vi "svx_Continuous Swept-Sine Waveform.vi"(10 "block size [samples]":i32, 11 "chirp settings":T1={"amplitude"=0.0, "frequency range"={"start (Hz)"=20.0, "stop (Hz)"=20000.0, "frequency spacing"=enum."Logarithmic"}, "sampling info"={"Fs"=50000.0, "chirp duration [s]"=3.0}, "initial states"={"frequency [Hz]"=20.0, "phase [rad]"=0.0, "elapsed time [s]"=0.0}, "frequency slope"=0.0, "maximum harmonic"=0, "prefix len [samples]"={"integer"=0, "fractional"=0.0}} {"frequency slope" format="%.2f"; "prefix len [samples]"."fractional" format="%.2p"; "initial states"."elapsed time [s]" format="%.2f"; "initial states"."phase [rad]" format="%.2f"; "initial states"."frequency [Hz]" format="%.2f"; "sampling info"."chirp duration [s]" format="%.2f"; "sampling info"."Fs" format="%.2p"; "frequency range"."stop (Hz)" format="%.2f"; "frequency range"."start (Hz)" format="%.2f"; "amplitude" format="%.2f"}) -> (1 "end reached?":bool, 2 "chirp signal":dbl[](array[numeric]), 3 "chirp settings out":T1={"amplitude"=0.0, "frequency range"={"start (Hz)"=20.0, "stop (Hz)"=20000.0, "frequency spacing"=enum."Logarithmic"}, "sampling info"={"Fs"=50000.0, "chirp duration [s]"=3.0}, "initial states"={"frequency [Hz]"=20.0, "phase [rad]"=0.0, "elapsed time [s]"=0.0}, "frequency slope"=0.0, "maximum harmonic"=0, "prefix len [samples]"={"integer"=0, "fractional"=0.0}} {"frequency slope" format="%.2f"; "prefix len [samples]"."fractional" format="%.2p"; "initial states"."elapsed time [s]" format="%.2f"; "initial states"."phase [rad]" format="%.2f"; "initial states"."frequency [Hz]" format="%.2f"; "sampling info"."chirp duration [s]" format="%.2f"; "sampling info"."Fs" format="%.2p"; "frequency range"."stop (Hz)" format="%.2f"; "frequency range"."start (Hz)" format="%.2f"; "amplitude" format="%.2f"})   [LabVIEW 2017]
uses:
  <vilib>/addons/_NISVFA/_Generation/subVIs/sv_Chirp Settings.ctl
  <vilib>/Analysis/1siggen.llb/Ramp Pattern by Samples.vi
  <vilib>/addons/_NISVFA/_Generation/SoundVib_Generation.lvlib
  <vilib>/Analysis/NI_AALBase.lvlib
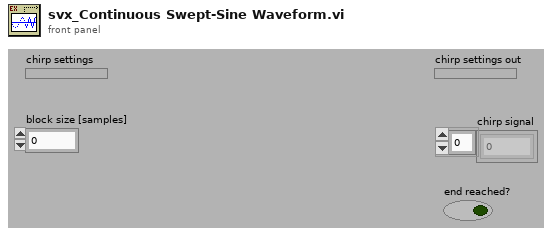
[diagram p1: front panel]
types:
  T1 = typedef "SoundVib_Generation.lvlib/sv_Chirp Settings.ctl" = cluster{"amplitude":dbl, "frequency range":cluster{"start (Hz)":dbl, "stop (Hz)":dbl, "frequency spacing":enum16{"Linear", "Logarithmic"}}, "sampling info":cluster{"Fs":dbl, "chirp duration [s]":dbl}, "initial states":cluster{"frequency [Hz]":dbl, "phase [rad]":dbl, "elapsed time [s]":dbl}, "frequency slope":dbl, "maximum harmonic":i32, "prefix len [samples]":cluster{"integer":u32, "fractional":dbl}}
  T2 = cluster{"frequency [Hz]":dbl, "phase [rad]":dbl, "elapsed time [s]":dbl}
  T3 = cluster{"start (Hz)":dbl, "stop (Hz)":dbl, "frequency spacing":enum16{"Linear", "Logarithmic"}}
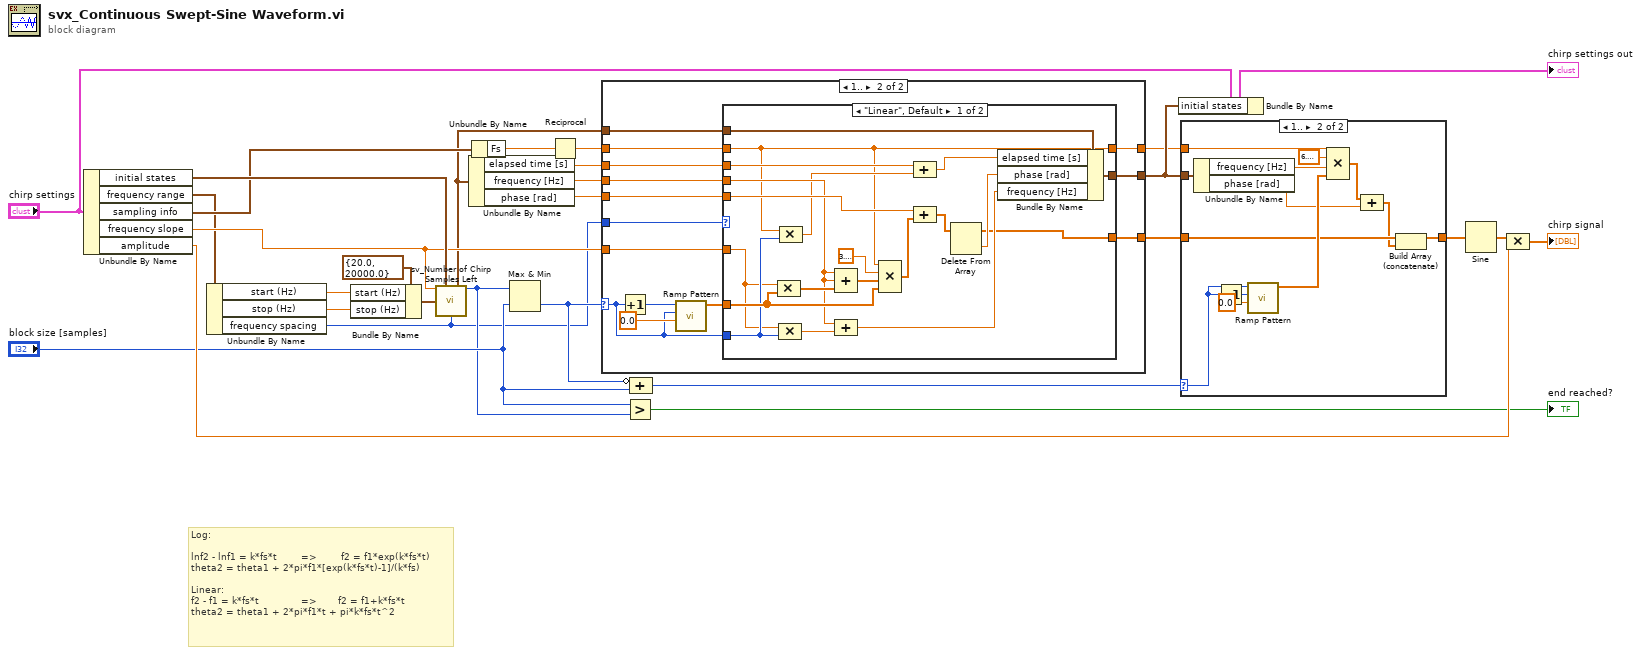
[diagram p0: block diagram]
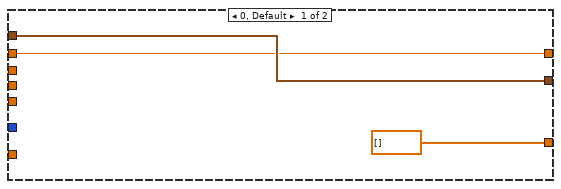
[diagram p2: hidden frame]
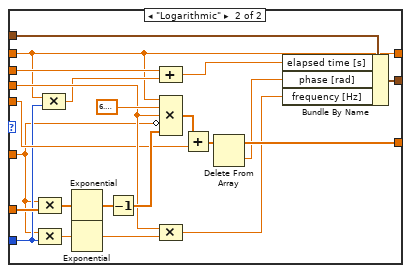
[diagram p3: hidden frame]
diagram:
  # "Log:\n            \nlnf2 - lnf1 = k*fs*t        =>        f2 = f1*exp(k*fs*t)\ntheta2 = theta1 + 2*pi*f1*[exp(k*fs*t)-1]/(k*fs)\n\nLinear:\nf2 - f1 = k*fs*t              =>       f2 = f1+k*fs*t\ntheta2 = theta1 + 2*pi*f1*t + pi*k*fs*t^2"
  n1 = Unbundle By Name("chirp settings") -> ("initial states"=w29:T2, "frequency range"=w9:T3, "sampling info"=w28:cluster{"Fs":dbl, "chirp duration [s]":dbl}, "frequency slope"=w27:dbl, "amplitude"=w15:dbl)
  n2 = Unbundle By Name(w9) -> ("start (Hz)"=w7:dbl, "stop (Hz)"=w6:dbl, "frequency spacing"=w1:enum16{"Linear", "Logarithmic"})
  n3 = Bundle By Name(cluster=cluster{"start (Hz)":dbl, "stop (Hz)":dbl} {"start (Hz)"=20.0, "stop (Hz)"=20000.0} ("frequency range"), "start (Hz)"=w7, "stop (Hz)"=w6) -> (w5:cluster{"start (Hz)":dbl, "stop (Hz)":dbl})
  n4 = call <vilib>:"sv_Number of Chirp Samples Left.vi"("frequency slope"=w27, "initial states"=w29, "frequency range"=w5, "frequency spacing"=w1) -> ("initial states out"=w22:T2, "# of samples left"=w3:i32)  [unwired: 9 in, 1 out]
  n5 = Unbundle By Name(w22) -> ("elapsed time [s]"=w23:dbl, "frequency [Hz]"=w26:dbl, "phase [rad]"=w25:dbl)
  n6 = Unbundle By Name(w28) -> ("Fs"=w24:dbl)
  n7 = Max & Min(x=w3, y="block size [samples]") -> (min(x,y)=w12:i32)  [unwired: 1 out]
  n8 = Reciprocal(x=w24) -> (1/x=w21:dbl)
  n9 = case shown="1.." w12 {
    selector: w12 -> [_ w33]
    tunnel: w27 -> [_ w46]
    tunnel: w26 -> [_ w45]
    tunnel: w25 -> [_ w44]
    tunnel: w1 -> [_ w40]
    tunnel: [dbl[] [] w39] -> w11
    tunnel: w23 -> [_ w38]
    tunnel: w22 -> [w32 w37]
    tunnel: w21 -> [w31 w36]
    tunnel: [w32 w35] -> w17
    tunnel: [w31 w34] -> w16
    frame 0, Default {
    }
    frame 1.. {
      n10 = Increment(x=w33) -> (x+1=w42:i32)
      n11 = call-poly <vilib>:"Ramp Pattern.vi"("start"=0.0, "end"=w33, "samples"=w42) -> ("Ramp Pattern"=w41:dbl[])  [unwired: 7 in, 1 out]
      n12 = case shown="\"Linear\", Default" w40 {
        tunnel: w45 -> [w56 w79]
        tunnel: w44 -> [w63 w76]
        tunnel: w46 -> [w48 w70]
        tunnel: w41 -> [w64 w84]
        tunnel: w37 -> [w49 w71]
        tunnel: w33 -> [w53 w75]
        tunnel: [w60 w78] -> w35
        tunnel: w36 -> [w47 w67]
        tunnel: [w54 w77] -> w39
        tunnel: w38 -> [w51 w73]
        tunnel: [w47 w67] -> w34
        frame "Linear", Default {
          n13 = Compound Arithmetic op=MULTIPLY(w48, w64) -> (w66:dbl[])
          n14 = Compound Arithmetic op=MULTIPLY(w48, w53) -> (w58:dbl)
          n15 = Compound Arithmetic op=MULTIPLY(w47, w53) -> (w52:dbl)
          n16 = Compound Arithmetic op=ADD(w56, w56, w66) -> (w65:dbl[])
          n17 = Compound Arithmetic op=ADD(w56, w58) -> (w57:dbl)
          n18 = Compound Arithmetic op=MULTIPLY(w47, 3.141592653589793, w65, w64) -> (w62:dbl[])
          n19 = Compound Arithmetic op=ADD(w51, w52) -> (w50:dbl)
          n20 = Compound Arithmetic op=ADD(w63, w62) -> (w61:dbl[])
          n21 = Delete From Array(array=w61) -> (deleted portion=w59:dbl, array with subset deleted=w54:dbl[])  [unwired: 2 in]
          n22 = Bundle By Name(cluster=w49, "elapsed time [s]"=w50, "phase [rad]"=w59, "frequency [Hz]"=w57) -> (w60:T2)
        }
        frame "Logarithmic" {
          n23 = Compound Arithmetic op=MULTIPLY(w70, w84) -> (w88:dbl[])
          n24 = Compound Arithmetic op=MULTIPLY(w70, w75) -> (w82:dbl)
          n25 = Compound Arithmetic op=MULTIPLY(w67, w75) -> (w74:dbl)
          n26 = Exponential(1:w88) -> (0:w83:dbl[])
          n27 = Exponential(1:w82) -> (0:w80:dbl)
          n28 = Decrement(x=w83) -> (x-1=w81:dbl[])
          n29 = Compound Arithmetic op=ADD(w73, w74) -> (w72:dbl)
          n30 = Compound Arithmetic op=MULTIPLY(w67, 6.283185307179586, w79, invert w70, w81) -> (w86:dbl[])
          n31 = Compound Arithmetic op=MULTIPLY(w79, w80) -> (w69:dbl)
          n32 = Add(x=w86, y=w76) -> (x+y=w85:dbl[])
          n33 = Delete From Array(array=w85) -> (deleted portion=w68:dbl, array with subset deleted=w77:dbl[])  [unwired: 2 in]
          n34 = Bundle By Name(cluster=w71, "elapsed time [s]"=w72, "phase [rad]"=w68, "frequency [Hz]"=w69) -> (w78:T2)
        }
      }
    }
  }
  n35 = Greater?(x="block size [samples]", y=w3) -> (0:→"end reached?":bool)
  n36 = Compound Arithmetic op=ADD(invert w12, "block size [samples]") -> (w18:i32)
  n37 = Bundle By Name(cluster="chirp settings", "initial states"=w17) -> (→"chirp settings out":T1)
  n38 = case shown="1.." w18 {
    selector: w18 -> [_ w90]
    tunnel: w17 -> [_ w102]
    tunnel: w16 -> [_ w97]
    tunnel: w11 -> [w89 w93]
    tunnel: [w89 w92] -> w14
    frame 0, Default {
    }
    frame 1.. {
      n39 = Unbundle By Name(w102) -> ("frequency [Hz]"=w98:dbl, "phase [rad]"=w94:dbl)
      n40 = Decrement(x=w90) -> (x-1=w101:i32)
      n41 = call-poly <vilib>:"Ramp Pattern.vi"("start"=0.0, "end"=w101, "samples"=w90) -> ("Ramp Pattern"=w99:dbl[])  [unwired: 7 in, 1 out]
      n42 = Compound Arithmetic op=MULTIPLY(w97, 6.283185307179586, w98, w99) -> (w95:dbl[])
      n43 = Compound Arithmetic op=ADD(w95, w94) -> (w91:dbl[])
      n44 = Build Array (concatenate)(w93, w91) -> (w92:dbl[])
    }
  }
  n45 = Sine(x=w14) -> (sin(x)=w10:dbl[])
  n46 = Compound Arithmetic op=MULTIPLY(w10, w15) -> (→"chirp signal":dbl[])
